vi "Init Interaction Splitter.vi"(6 "user event out":refnum<user-event>, 7 "Vertical? [F]":bool, 8 "error in (no error)":errorcluster, 10 "Host VI":refnum<vi>) -> (0 "error out":errorcluster, 3 "Interaction Splitter out":refnum<class "Interaction Splitter.lvclass">)   [LabVIEW 2021, in "Interaction Splitter.lvclass"]
doc: "Copyright 2018, Wiebe Walstra, wiebe@carya.nl."
uses:
  Interaction Splitter.lvclass
  Interaction Splitter.lvclass/Interaction Splitter.ctl
  Dynamic Event Handler.vi
  Vertical Splitter.vi
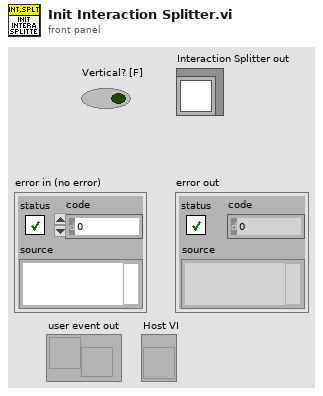
[diagram p1: front panel]
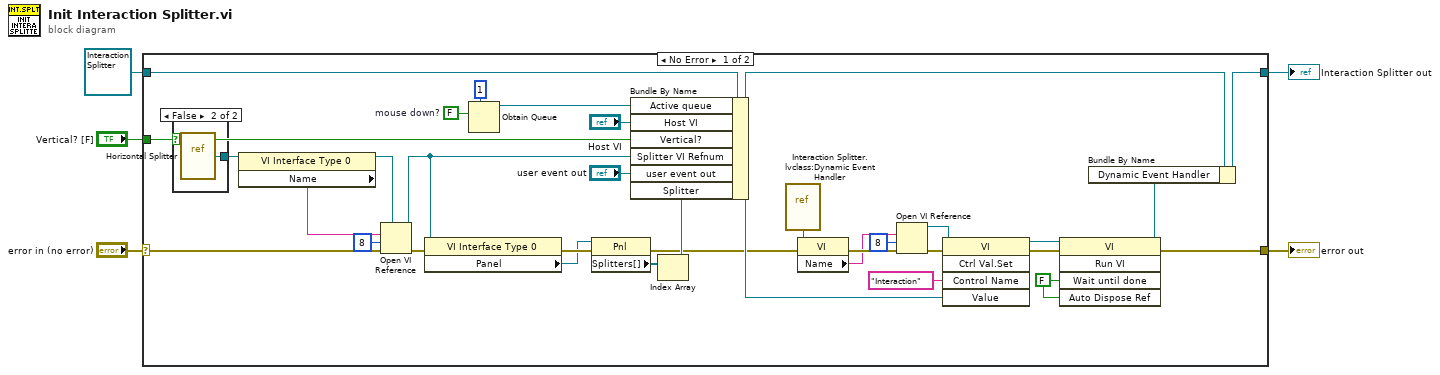
[diagram p0: block diagram]
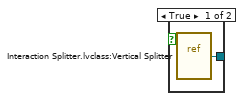
[diagram p2: hidden frame]
diagram:
  n1 = case shown="No Error" "error in (no error)" {
    selector: "error in (no error)" -> [w32 w41]
    tunnel: [w10 w41] -> w4
    tunnel: [w17 w40] -> w2
    tunnel: refnum<class "Interaction Splitter.lvclass"> refnum ("Interaction Splitter in") -> [w34 w40]
    tunnel: "Vertical? [F]" -> [w33 _]
    frame No Error {
      w8 = FALSE  # mouse down?
      w26 = FALSE ("Wait Until Done")
      n2 = case shown="False" w33 {
        tunnel: [w38 w39] -> w31
        frame True {
          n3 = vi-ref "Interaction Splitter.lvclass:Vertical Splitter.vi"() -> (w38:refnum<vi>)
        }
        frame False {
          n4 = vi-ref "Horizontal Splitter.vi"() -> (w39:refnum<vi>)
        }
      }
      n5 = property class="VI Interface Type 0"(reference=w31) -> (reference out=w29:refnum<vi>, "Name"=w30:string)  [unwired: 1 in, 1 out]
      n6 = Open VI Reference(type specifier VI Refnum (for type only)=w29, vi path=w30, options=8, error in (no error)=w32) -> (vi reference=w13:refnum<vi>, error out=w14:errorcluster)  [unwired: 2 in]
      n7 = property class="VI Interface Type 0"(reference=w13, error in=w14) -> (error out=w36:errorcluster, "Panel"=w35:refnum<vi>)  [unwired: 1 out]
      n8 = Obtain Queue(max queue size (-1, unlimited)=1, element data type=w8) -> (queue out=w6:refnum<queue>)  [unwired: 3 in, 2 out]
      n9 = property class="Pnl"(reference=w35, error in=w36) -> (error out=w11:errorcluster, "Splitters[]"=w37:refnum<vi>[])  [unwired: 1 out]
      n10 = Index Array(array=w37) -> (element=w12:refnum<vi>)  [unwired: 1 in]
      n11 = Bundle By Name(cluster=w34, "Active queue"=w6, "Host VI"="Host VI", "Vertical?"=w33, "Splitter VI Refnum"=w13, "user event out"="user event out", "Splitter"=w12) -> (w16:refnum<class "Interaction Splitter.lvclass">)
      n12 = vi-ref "Interaction Splitter.lvclass:Dynamic Event Handler.vi"() -> (w18:refnum<vi>)
      n13 = property class="VI"(reference=w18, error in=w11) -> (error out=w21:errorcluster, "Name"=w19:string)  [unwired: 1 out]
      n14 = Open VI Reference(vi path=w19, options=8, error in (no error)=w21) -> (vi reference=w23:refnum<vi>)  [unwired: 3 in, 1 out]
      n15 = invoke class="VI" method="Ctrl Val.Set"(reference=w23, error in=w21, "Control Name"="Interaction", "Value"=w16) -> (reference out=w24:refnum<vi>, error out=w22:errorcluster)  [unwired: 1 in, 3 out]
      n16 = invoke class="VI" method="Run VI"(reference=w24, error in=w22, "Wait until done"=w26, "Auto Dispose Ref"=w26) -> (reference out=w25:refnum<vi>, error out=w10:errorcluster)  [unwired: 1 in, 3 out]
      n17 = Bundle By Name(cluster=w16, "Dynamic Event Handler"=w25) -> (w17:refnum<class "Interaction Splitter.lvclass">)
    }
    frame Error {
    }
  }
  "error out" <- w4
  "Interaction Splitter out" <- w2
